vi "dR_R_ForFile.vi"(6 "DR/R parameter":T1={"frame_zero_0"=0, "frame_zero_1"=1, "frame_0"=3, "frame_1"=15}, 7 "clip ratio":dbl=2.0, 8 "stim ID":u8[](array[numeric])=[0, 2, 4, 6, 8], 9 "OnlineMap":cluster{"数组 1":i32[], "数组 2":i32[]}[](array[cluster])=[{"数组 1"=[2], "数组 2"=[6]}, {"数组 1"=[4], "数组 2"=[8]}, {"数组 1"=[2, 6], "数组 2"=[4, 8]}, {"数组 1"=[2, 4, 6, 8], "数组 2"=[0]}, {"数组 1"=[2, 4], "数组 2"=[6, 8]}], 10 "blkIndex":i32, 11 "BlkFile":refnum<file>) -> (3 "onLineMapOutput":T2[](array[typedef]))   [LabVIEW 2011]
uses:
  <vilib>/vision/Image Controls.llb/IMAQ Image.ctl
  <vilib>/vision/NI_Vision_Development_Module.lvlib
  <vilib>/Analysis/NI_AALBase.lvlib
panel:
  in  "选项卡控件":enum32{"选项卡 1", "选项卡 2"}(tab)
  out "datatype":u16(ring)=13 items=["U8"=11, "I16"=12, "U32"=13, "SGL"=14]
  out "FramesPerStim(100Hz)":i64=16
  out "FrameWidth":i64=704
  out "FrameHeight":i64=576
  out "OnlineMap Array":T2[](array[typedef])
  # "÷"
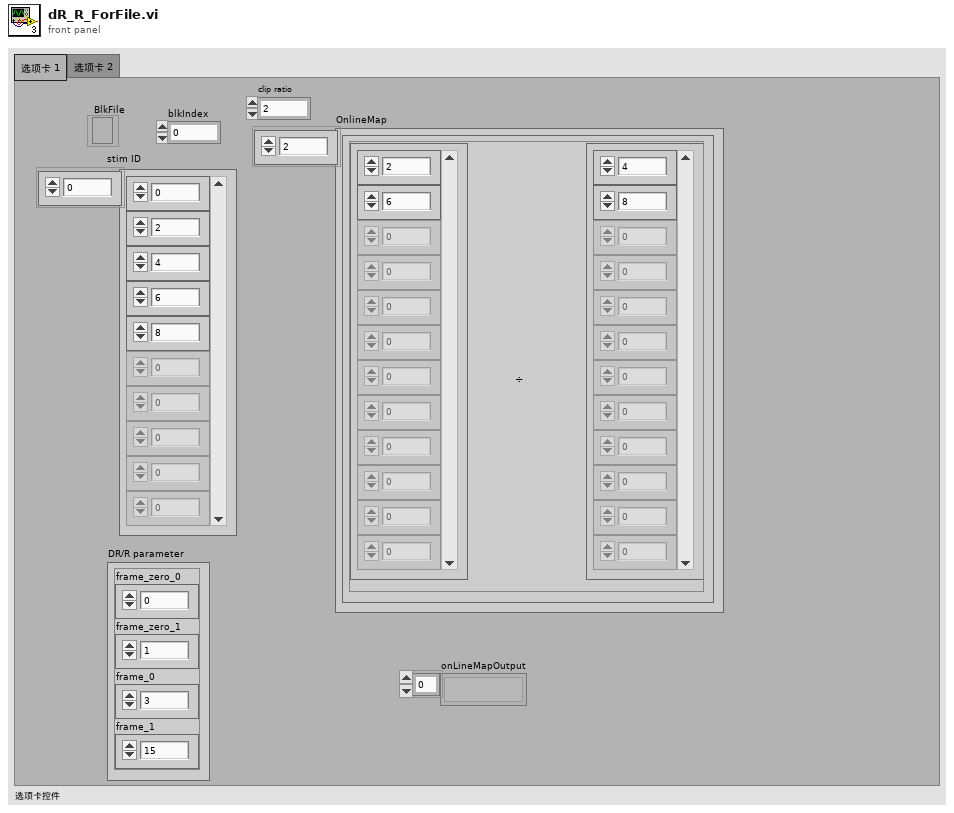
[diagram p1: front panel]
types:
  T1 = cluster{"frame_zero_0":i32, "frame_zero_1":i32, "frame_0":i32, "frame_1":i32}
  T2 = typedef "IMAQ Image.ctl" = refnum<image>
  T3 = enum16{"big-endian, network order", "native, host order", "little-endian"}
  T4 = typedef "Image Type" = u32
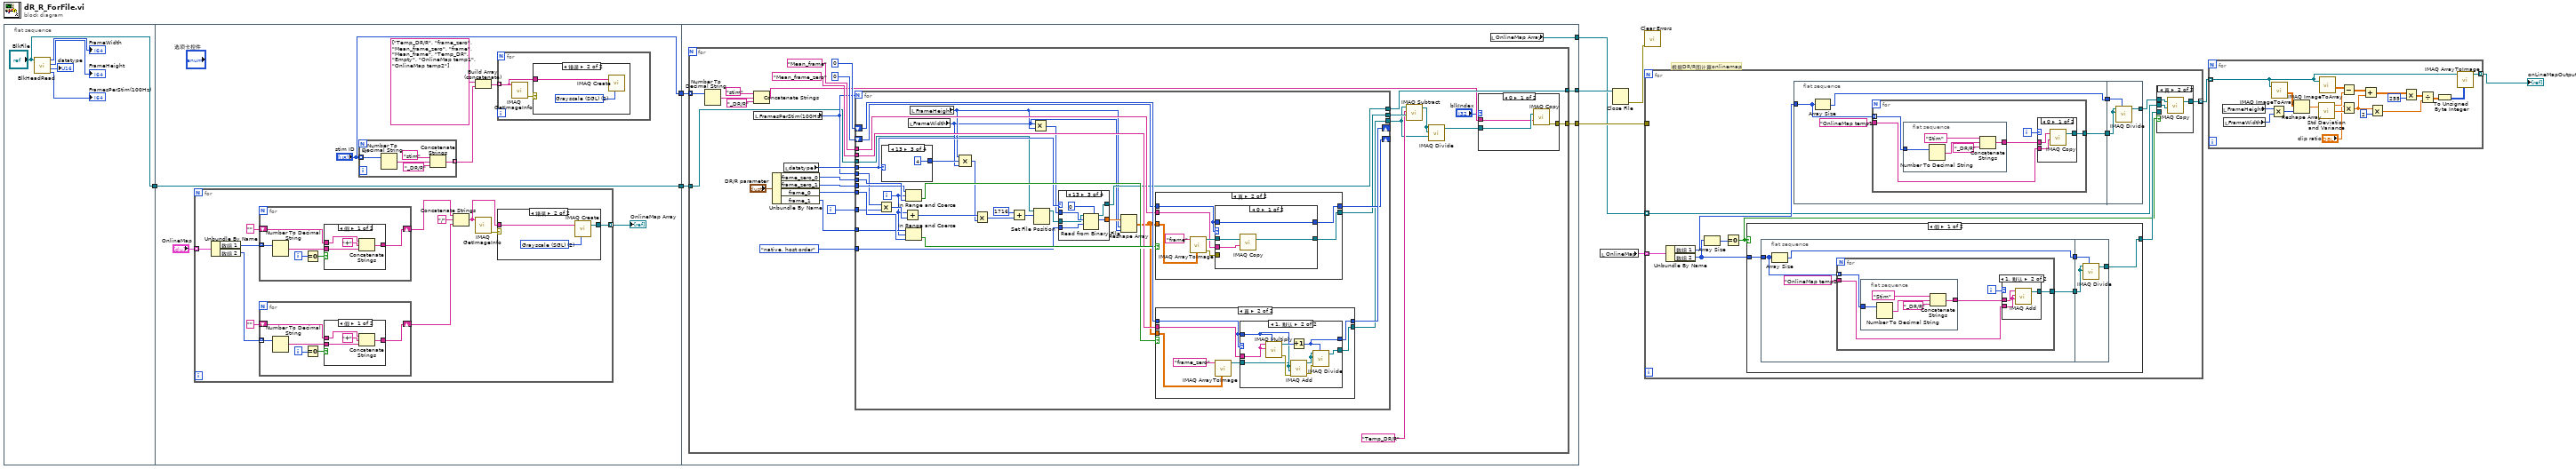
[diagram p0: block diagram]
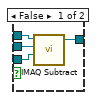
[diagram p2: hidden frame]
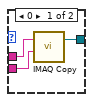
[diagram p3: hidden frame]
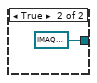
[diagram p4: hidden frame]
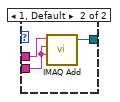
[diagram p5: hidden frame]
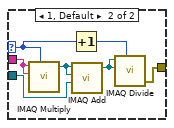
[diagram p10: hidden frame]
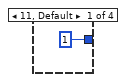
[diagram p11: hidden frame]
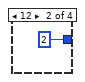
[diagram p12: hidden frame]
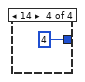
[diagram p13: hidden frame]
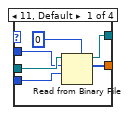
[diagram p14: hidden frame]
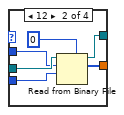
[diagram p15: hidden frame]
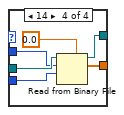
[diagram p16: hidden frame]
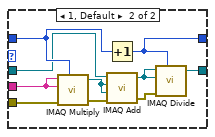
[diagram p18: hidden frame]
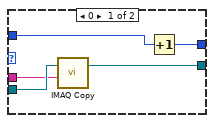
[diagram p20: hidden frame]
diagram:
  # "根据DR/R图计算onlinemap"
  n1 = flat-sequence {
    tunnel: ["BlkFile"] -> w10
    tunnel: ["stim ID"] -> w9
    tunnel: [w22] -> w8
    tunnel: w10 -> [w22]
    tunnel: [w73] -> w6
    tunnel: [w72] -> w5
    tunnel: w9 -> [w71]
    tunnel: w8 -> [w70]
    tunnel: [w69] -> w1
    frame #0 {
      n2 = call "BlkHeadRead.vi"("引用句柄"="BlkFile") -> ("FramesPerStim"=→"FramesPerStim(100Hz)":i32, "datatype"=→"datatype":i32, "FrameHeight"=→"FrameHeight":i32, "FrameWidth"=→"FrameWidth":i32)  [unwired: 5 in, 2 out]
    }
    frame #1 {
      n3 = for {
        tunnel: "OnlineMap" -> [w38] mode=indexing
        tunnel: [w29] -> w20 mode=indexing
        n4 = Unbundle By Name(w38) -> ("数组 1"=w37:i32[], "数组 2"=w34:i32[])
        n5 = for {
          tunnel: w37 -> [w57] mode=indexing
          shift-right: [w55] -> w35
          shift-left: "" -> [w54]
          i -> [w59]
          n6 = Number To Decimal String(number=w57) -> (decimal integer string=w56:string)  [unwired: 1 in]
          n7 = Equal To 0?(x=w59) -> (x = 0?=w58:bool)
          n8 = case shown="假" w58 {
            tunnel: w56 -> [w60 w64]
            tunnel: [w63 w64] -> w55
            tunnel: w54 -> [w62 _]
            frame False {
              n9 = Concatenate Strings(w62, "+" ("字符串"), w60) -> (w63:string)
            }
            frame True {
            }
          }
        }
        n10 = for {
          tunnel: w34 -> [w46] mode=indexing
          shift-right: [w44] -> w32
          shift-left: "" -> [w43]
          i -> [w48]
          n11 = Number To Decimal String(number=w46) -> (decimal integer string=w45:string)  [unwired: 1 in]
          n12 = Equal To 0?(x=w48) -> (x = 0?=w47:bool)
          n13 = case shown="假" w47 {
            tunnel: w45 -> [w49 w53]
            tunnel: [w52 w53] -> w44
            tunnel: w43 -> [w51 _]
            frame False {
              n14 = Concatenate Strings(w51, "+" ("字符串"), w49) -> (w52:string)
            }
            frame True {
            }
          }
        }
        n15 = Concatenate Strings(w35, "/" ("字符串"), w32) -> (w28:string)
        n16 = call "IMAQ GetImageInfo"("Image"=w28) -> ("error out"=w30:errorcluster)  [unwired: 3 in, 7 out]
        n17 = case shown="错误" w30 {
          tunnel: w28 -> [w39 w41]
          tunnel: [w39 w40] -> w29
          frame No Error {
          }
          frame Error {
            w42 = T4 2 items=["Grayscale (U8)", "Grayscale (I16)", "Grayscale (SGL)", "Complex (CSG)", "RGB (U32)", "HSL (U32)", "RGB (U64)", "Grayscale (U16)"] ("Image Type")
            n18 = call "IMAQ Create"("Image Name"=w41, "Image Type"=w42) -> ("New Image"=w40:T2)  [unwired: 3 in, 1 out]
          }
        }
      }
      "OnlineMap Array" <- w20
      n19 = for {
        tunnel: "stim ID" -> [w24] mode=indexing
        tunnel: [w23] -> w17 mode=indexing
        n20 = Number To Decimal String(number=w24) -> (decimal integer string=w25:string)  [unwired: 1 in]
        n21 = Concatenate Strings("stim" ("字符串"), w25, "_DR/R" ("字符串")) -> (w23:string)
      }
      n22 = Build Array (concatenate)(string[] ["Temp_DR/R", "frame_zero", "Mean_frame_zero", "frame", "Mean_frame", "Temp_DR", "Empty", "OnlineMap temp1", "OnlineMap temp2"] ("添加的数组"), w17) -> (w16:string[])
      n23 = for {
        tunnel: w16 -> [w65] mode=indexing
        n24 = call "IMAQ GetImageInfo"("Image"=w65) -> ("error out"=w66:errorcluster)  [unwired: 3 in, 7 out]
        n25 = case shown="错误" w66 {
          tunnel: w65 -> [_ w67]
          frame No Error {
          }
          frame Error {
            w68 = T4 2 items=["Grayscale (U8)", "Grayscale (I16)", "Grayscale (SGL)", "Complex (CSG)", "RGB (U32)", "HSL (U32)", "RGB (U64)", "Grayscale (U16)"] ("Image Type")
            n26 = call "IMAQ Create"("Image Name"=w67, "Image Type"=w68) -> ()  [unwired: 3 in, 2 out]
          }
        }
      }
    }
    frame #2 {
      n27 = for {
        tunnel: w71 -> [w80] mode=indexing
        tunnel: [w99] -> w73
        tunnel: [w86] -> w72
        tunnel: w70 -> [w78]
        i -> [w84]
        n28 = Number To Decimal String(number=w80) -> (decimal integer string=w83:string)  [unwired: 1 in]
        n29 = Concatenate Strings("stim" ("字符串"), w83, "_DR/R" ("字符串")) -> (w79:string)
        n30 = local read "FramesPerStim(100Hz)"() -> (w85:i64)
        n31 = Unbundle By Name("DR/R parameter") -> ("frame_zero_0"=w98:i32, "frame_zero_1"=w97:i32, "frame_0"=w95:i32, "frame_1"=w94:i32)
        n32 = local read "datatype"() -> (w87:u16)
        n33 = for {
          N: w85 -> [_]
          tunnel: w98 -> [w138]
          tunnel: w97 -> [w137]
          shift-right: [w143] -> _
          shift-left: 0 -> [w144]
          tunnel: w95 -> [w136]
          tunnel: w94 -> [w135]
          shift-right: [w141] -> _
          shift-left: 0 -> [w142]
          tunnel: "Mean_frame_zero" ("Image Name") -> [w133]
          tunnel: [w134] -> w77
          tunnel: "Mean_frame" ("Image Name") -> [w131]
          tunnel: [w132] -> w100
          tunnel: T3."native, host order" ("字节顺序(0:big-endian, network order)") -> [w129]
          tunnel: w87 -> [w126]
          tunnel: [w127] -> w86
          tunnel: w84 -> [w121]
          tunnel: w85 -> [w120]
          tunnel: w78 -> [w112]
          i -> [w118]
          n34 = Multiply(x=w120, y=w121) -> (x*y=w119:i64)
          n35 = case shown="13" w126 {
            tunnel: [i64 1 i64 2 i64 4 i64 4] -> w123
            frame 11, Default {
            }
            frame 12 {
            }
            frame 13 {
            }
            frame 14 {
            }
          }
          n36 = Add(x=w118, y=w119) -> (x+y=w117:i64)
          n37 = In Range and Coerce(upper limit=w137, x=w118, lower limit=w138) -> (In Range?=w139:bool)  [unwired: 1 out]
          n38 = In Range and Coerce(upper limit=w135, x=w118, lower limit=w136) -> (In Range?=w140:bool)  [unwired: 1 out]
          n39 = local read "FrameWidth"() -> (w122:i64)
          n40 = local read "FrameHeight"() -> (w124:i64)
          n41 = Compound Arithmetic op=MULTIPLY(w124, w123, w122) -> (w116:i64)
          n42 = Multiply(x=w117, y=w116) -> (x*y=w115:i64)
          n43 = Add(x=i64 1716, y=w115) -> (x+y=w113:i64)
          n44 = Multiply(x=w122, y=w124) -> (x*y=w125:i64)
          n45 = Set File Position(offset (in bytes) (0)=w113, refnum=w112) -> (refnum out=w130:refnum<file>)  [unwired: 2 in, 1 out]
          n46 = case shown="13" w126 {
            tunnel: w130 -> [w154 w159 w163 w171]
            tunnel: w125 -> [w153 w158 w165 w170]
            tunnel: w129 -> [w152 w157 w164 w169]
            tunnel: [w150 w156 w162 w168] -> w128
            tunnel: [w149 w155 w161 w167] -> w127
            frame 11, Default {
              n47 = Read from Binary File(5:u8 0, 9:w152, 10:w153, 11:w154) -> (2:w150:u8[], 3:w149:refnum<file>)  [unwired: 2 in, 2 out]
            }
            frame 12 {
              n48 = Read from Binary File(5:u16 0, 9:w157, 10:w158, 11:w159) -> (2:w156:u16[], 3:w155:refnum<file>)  [unwired: 2 in, 2 out]
            }
            frame 13 {
              n49 = Read from Binary File(5:u32 0, 9:w164, 10:w165, 11:w163) -> (2:w162:u32[], 3:w161:refnum<file>)  [unwired: 2 in, 2 out]
            }
            frame 14 {
              n50 = Read from Binary File(5:sgl 0.0, 9:w169, 10:w170, 11:w171) -> (2:w168:sgl[], 3:w167:refnum<file>)  [unwired: 2 in, 2 out]
            }
          }
          n51 = Reshape Array(w128, w124, w122) -> (w111:sgl[][])
          n52 = case shown="真" w140 {
            tunnel: w111 -> [_ w182]
            tunnel: w142 -> [w174 w175]
            tunnel: [w174 w178] -> w141
            tunnel: [w173 w177] -> w132
            tunnel: w131 -> [w173 w176]
            frame False {
            }
            frame True {
              n53 = call "IMAQ ArrayToImage"("Image Pixels (Float)"=w182, "Image"="frame" ("Image Name")) -> ("error out"=w179:errorcluster, "Image Out"=w180:T2)  [unwired: 8 in]
              n54 = case shown="0" w175 {
                tunnel: w175 -> [w183 w196]
                tunnel: w180 -> [w186 w195]
                tunnel: w179 -> [_ w191]
                tunnel: [w183 w190] -> w178
                tunnel: [w184 w188] -> w177
                tunnel: w176 -> [w185 w187]
                frame 0 {
                  n55 = call "IMAQ Copy"("Image Dst"=w185, "Image Src"=w186) -> ("Image Dst Out"=w184:T2)  [unwired: 4 in, 1 out]
                }
                frame 1, Default {
                  n56 = call "IMAQ Multiply"("Image Src A"=w187, "Constant"=w196, "Image Dst"=w187, "error in (no error)"=w191) -> ("Image Dst Out"=w194:T2, "error out"=w192:errorcluster)  [unwired: 3 in]
                  n57 = Increment(x=w196) -> (x+1=w190:i32)
                  n58 = call "IMAQ Add"("Image Src A"=w195, "Image Dst"=w194, "Image Src B"=w194, "error in (no error)"=w192) -> ("Image Dst Out"=w189:T2, "error out"=w193:errorcluster)  [unwired: 3 in]
                  n59 = call "IMAQ Divide"("Image Src A"=w189, "Constant"=w190, "Image Dst"=w189, "error in (no error)"=w193) -> ("Image Dst Out"=w188:T2)  [unwired: 3 in, 1 out]
                }
              }
            }
          }
          n60 = case shown="真" w139 {
            tunnel: w111 -> [_ w200]
            tunnel: w144 -> [w198 w202]
            tunnel: [w198 w205] -> w143
            tunnel: [w197 w204] -> w134
            tunnel: w133 -> [w197 w203]
            frame False {
            }
            frame True {
              n61 = call "IMAQ ArrayToImage"("Image Pixels (Float)"=w200, "Image"="frame_zero" ("Image Name")) -> ("Image Out"=w199:T2)  [unwired: 8 in, 1 out]
              n62 = case shown="1, 默认" w202 {
                tunnel: w202 -> [w207 w219]
                tunnel: [w206 w216] -> w205
                tunnel: w199 -> [w210 w213]
                tunnel: [w208 w212] -> w204
                tunnel: w203 -> [w209 w211]
                frame 0 {
                  n63 = call "IMAQ Copy"("Image Dst"=w209, "Image Src"=w210) -> ("Image Dst Out"=w208:T2)  [unwired: 4 in, 1 out]
                  n64 = Increment(x=w207) -> (x+1=w206:i32)
                }
                frame 1, Default {
                  n65 = call "IMAQ Multiply"("Image Src A"=w211, "Constant"=w219, "Image Dst"=w211) -> ("Image Dst Out"=w214:T2, "error out"=w217:errorcluster)  [unwired: 4 in]
                  n66 = Increment(x=w219) -> (x+1=w216:i32)
                  n67 = call "IMAQ Add"("Image Src A"=w213, "Image Dst"=w214, "Image Src B"=w214, "error in (no error)"=w217) -> ("Image Dst Out"=w215:T2, "error out"=w218:errorcluster)  [unwired: 3 in]
                  n68 = call "IMAQ Divide"("Image Src A"=w215, "Constant"=w216, "Image Dst"=w215, "error in (no error)"=w218) -> ("Image Dst Out"=w212:T2)  [unwired: 3 in, 1 out]
                }
              }
            }
          }
        }
        n69 = call "IMAQ Subtract"("Image Src A"=w77, "Image Dst"="Temp_DR/R" ("Image Name"), "Image Src B"=w100) -> ("Image Dst Out"=w76:T2)  [unwired: 4 in, 1 out]
        n70 = call "IMAQ Divide"("Image Src A"=w76, "Image Dst"=w76, "Image Src B"=w77) -> ("Image Dst Out"=w75:T2)  [unwired: 4 in, 1 out]
        n71 = case shown="0" "blkIndex" {
          selector: "blkIndex" -> [_ w107]
          tunnel: w75 -> [w103 w108]
          tunnel: w79 -> [w102 w110]
          tunnel: [w101 w104] -> w99
          frame 0 {
            n72 = call "IMAQ Copy"("Image Dst"=w102, "Image Src"=w103) -> ("error out"=w101:errorcluster)  [unwired: 4 in, 1 out]
          }
          frame 1, Default {
            n73 = call "IMAQ Multiply"("Image Src A"=w110, "Constant"=w107, "Image Dst"=w110) -> ("Image Dst Out"=w109:T2)  [unwired: 4 in, 1 out]
            n74 = Increment(x=w107) -> (x+1=w106:i32)
            n75 = call "IMAQ Add"("Image Src A"=w109, "Image Dst"=w109, "Image Src B"=w108) -> ("Image Dst Out"=w105:T2)  [unwired: 4 in, 1 out]
            n76 = call "IMAQ Divide"("Image Src A"=w105, "Constant"=w106, "Image Dst"=w105) -> ("error out"=w104:errorcluster)  [unwired: 4 in, 1 out]
          }
        }
      }
      n77 = local read "OnlineMap Array"() -> (w69:T2[])
    }
  }
  n78 = local read "OnlineMap"() -> (w4:cluster{"数组 1":i32[], "数组 2":i32[]}[])
  n79 = Close File(refnum=w5) -> (error out=w7:errorcluster)  [unwired: 1 in, 1 out]
  n80 = call <vilib>:"Clear Errors.vi"("error in (no error)"=w7) -> ()  [unwired: 6 in, 1 out]
  n81 = for {
    tunnel: w4 -> [w230] mode=indexing
    tunnel: w1 -> [w226] mode=indexing
    tunnel: [w223] -> w3 mode=indexing
    tunnel: w6 -> [_]
    n82 = Unbundle By Name(w230) -> ("数组 1"=w229:i32[], "数组 2"=w221:i32[])
    n83 = Array Size(array=w221) -> (size(s)=w222:i32)
    n84 = Equal To 0?(x=w222) -> (x = 0?=w220:bool)
    n85 = case shown="假" w220 {
      tunnel: [w239 T2 refnum ("Image Dst Out")] -> w224
      tunnel: w221 -> [w238 _]
      frame False {
        n86 = flat-sequence {
          tunnel: w238 -> [w242]
          tunnel: [w244] -> w241
          tunnel: [w243] -> w240
          tunnel: w241 -> [w263]
          tunnel: w240 -> [w264]
          tunnel: [w262] -> w239
          frame #0 {
            n87 = Array Size(array=w242) -> (size(s)=w243:i32)
            n88 = for {
              tunnel: w242 -> [w250] mode=indexing
              tunnel: "OnlineMap temp2" ("Image Name") -> [w248]
              tunnel: [w246] -> w244
              i -> [w247]
              n89 = flat-sequence {
                tunnel: w250 -> [w259]
                tunnel: [w257] -> w249
                frame #0 {
                  n90 = Number To Decimal String(number=w259) -> (decimal integer string=w260:string)  [unwired: 1 in]
                  n91 = Concatenate Strings("Stim", w260, "_DR/R" ("字符串")) -> (w257:string)
                }
              }
              n92 = case shown="1, 默认" w247 {
                tunnel: w249 -> [w253 w256]
                tunnel: w248 -> [w252 w255]
                tunnel: [w251 w254] -> w246
                frame 0 {
                  n93 = call "IMAQ Copy"("Image Dst"=w252, "Image Src"=w253) -> ("Image Dst Out"=w251:T2)  [unwired: 4 in, 1 out]
                }
                frame 1, Default {
                  n94 = call "IMAQ Add"("Image Src A"=w256, "Image Dst"=w255, "Image Src B"=w255) -> ("Image Dst Out"=w254:T2)  [unwired: 4 in, 1 out]
                }
              }
            }
          }
          frame #1 {
            n95 = call "IMAQ Divide"("Image Src A"=w263, "Constant"=w264, "Image Dst"=w263) -> ("Image Dst Out"=w262:T2)  [unwired: 4 in, 1 out]
          }
        }
      }
      frame True {
      }
    }
    n96 = flat-sequence {
      tunnel: w229 -> [w268]
      tunnel: [w267] -> w228
      tunnel: [w266] -> w227
      tunnel: w228 -> [w287]
      tunnel: w227 -> [w288]
      tunnel: [w286] -> w225
      frame #0 {
        n97 = Array Size(array=w268) -> (size(s)=w266:i32)
        n98 = for {
          tunnel: w268 -> [w274] mode=indexing
          tunnel: "OnlineMap temp1" ("Image Name") -> [w272]
          tunnel: [w270] -> w267
          i -> [w271]
          n99 = flat-sequence {
            tunnel: w274 -> [w283]
            tunnel: [w281] -> w273
            frame #0 {
              n100 = Number To Decimal String(number=w283) -> (decimal integer string=w284:string)  [unwired: 1 in]
              n101 = Concatenate Strings("Stim", w284, "_DR/R" ("字符串")) -> (w281:string)
            }
          }
          n102 = case shown="0" w271 {
            tunnel: w273 -> [w277 w280]
            tunnel: w272 -> [w276 w279]
            tunnel: [w275 w278] -> w270
            frame 0 {
              n103 = call "IMAQ Copy"("Image Dst"=w276, "Image Src"=w277) -> ("Image Dst Out"=w275:T2)  [unwired: 4 in, 1 out]
            }
            frame 1, Default {
              n104 = call "IMAQ Add"("Image Src A"=w280, "Image Dst"=w279, "Image Src B"=w279) -> ("Image Dst Out"=w278:T2)  [unwired: 4 in, 1 out]
            }
          }
        }
      }
      frame #1 {
        n105 = call "IMAQ Divide"("Image Src A"=w287, "Constant"=w288, "Image Dst"=w287) -> ("Image Dst Out"=w286:T2)  [unwired: 4 in, 1 out]
      }
    }
    n106 = case shown="真" w220 {
      tunnel: w226 -> [w234 w236]
      tunnel: w225 -> [w233 w237]
      tunnel: w224 -> [w232 _]
      tunnel: [w231 w235] -> w223
      frame False {
        n107 = call "IMAQ Subtract"("Image Src A"=w233, "Image Dst"=w234, "Image Src B"=w232) -> ("Image Dst Out"=w231:T2)  [unwired: 4 in, 1 out]
      }
      frame True {
        n108 = call "IMAQ Copy"("Image Dst"=w236, "Image Src"=w237) -> ("Image Dst Out"=w235:T2)  [unwired: 4 in, 1 out]
      }
    }
  }
  n109 = for {
    tunnel: w3 -> [w304] mode=indexing
    tunnel: [w303] -> w2 mode=indexing
    n110 = local read "FrameHeight"() -> (w299:i64)
    n111 = local read "FrameWidth"() -> (w298:i64)
    n112 = Multiply(x=w299, y=w298) -> (x*y=w300:i64)
    n113 = call "IMAQ ImageToArray"("Image"=w304) -> ("Image Pixels (Float)"=w301:sgl[][])  [unwired: 3 in, 4 out]
    n114 = Reshape Array(w301, w300) -> (w305:sgl[])
    n115 = call <vilib>:"Std Deviation and Variance.vi"("X"=w305) -> ("mean"=w297:dbl, "standard deviation"=w295:dbl)  [unwired: 1 in, 1 out]
    n116 = call "IMAQ ImageToArray"("Image"=w304) -> ("Image Pixels (Float)"=w306:sgl[][])  [unwired: 3 in, 4 out]
    n117 = Subtract(x=w306, y=w297) -> (x-y=w296:dbl[][])
    n118 = Multiply(x="clip ratio", y=w295) -> (x*y=w290:dbl)
    n119 = Add(x=w296, y=w290) -> (x+y=w294:dbl[][])
    n120 = Multiply(x=w290, y=2) -> (x*y=w289:dbl)
    n121 = Multiply(x=w294, y=255) -> (x*y=w293:dbl[][])
    n122 = Divide(x=w293, y=w289) -> (x/y=w292:dbl[][])
    n123 = To Unsigned Byte Integer(number=w292) -> (unsigned 8bit integer=w302:u8[][])
    n124 = call "IMAQ ArrayToImage"("Image Pixels (Float)"=w302, "Image"=w304) -> ("Image Out"=w303:T2)  [unwired: 8 in, 1 out]
  }
  "onLineMapOutput" <- w2
